vi "Frequency Sweeper Sub VI (FINAL).vi"(1 "Numeric":dbl, 2 "error in (no error)":errorcluster, 3 "VISA resource name":refnum<visa-resource-name>="USB0::0x0699::0x0353::1612076::INSTR") -> (0 "error out":errorcluster)   [LabVIEW 2017]
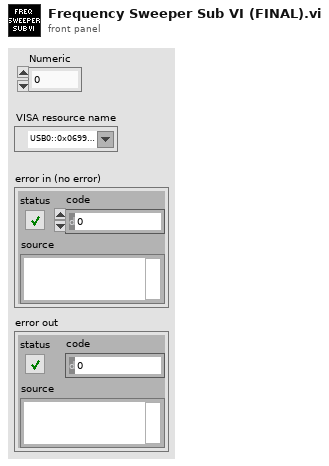
[diagram p1: front panel]
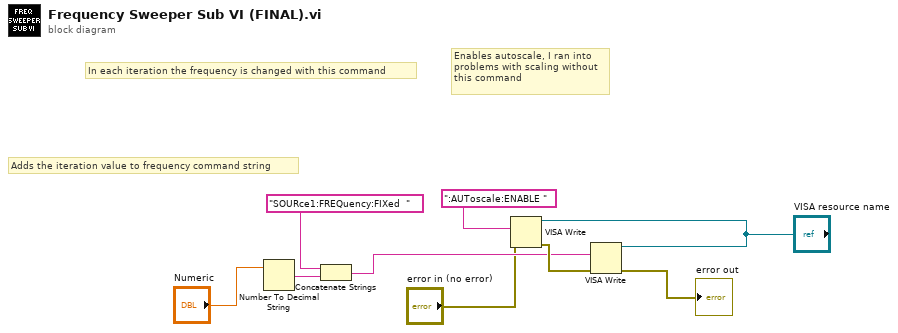
[diagram p0: block diagram]
diagram:
  # "Adds the iteration value to frequency command string"
  # "Enables autoscale, I ran into problems with scaling without this command"
  # "In each iteration the frequency is changed with this command"
  n1 = Number To Decimal String(number="Numeric") -> (decimal integer string=w3:string)  [unwired: 1 in]
  n2 = Concatenate Strings("SOURce1:FREQuency:FIXed  " ("write buffer"), w3) -> (w5:string)
  n3 = VISA Write(VISA resource name="VISA resource name", write buffer=":AUToscale:ENABLE ", error in (no error)="error in (no error)") -> (error out=w8:errorcluster)  [unwired: 2 out]
  n4 = VISA Write(VISA resource name="VISA resource name", write buffer=w5, error in (no error)=w8) -> (error out=→"error out":errorcluster)  [unwired: 2 out]
